vi "Moving Average.vi"(9 "New Value":dbl, 10 "# of Previous Elements":u64, 11 "Previous Average":dbl) -> (2 "Average":dbl)   [LabVIEW 2016]
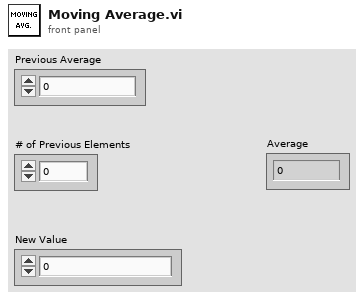
[diagram p1: front panel]
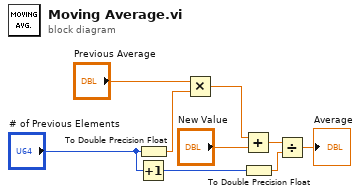
[diagram p0: block diagram]
diagram:
  n1 = Increment(x="# of Previous Elements") -> (x+1=w2:u64)
  n2 = To Double Precision Float(number="# of Previous Elements") -> (double precision float=w3:dbl)
  n3 = Multiply(x="Previous Average", y=w3) -> (x*y=w8:dbl)
  n4 = Add(x=w8, y="New Value") -> (x+y=w6:dbl)
  n5 = To Double Precision Float(number=w2) -> (double precision float=w1:dbl)
  n6 = Divide(x=w6, y=w1) -> (x/y=→"Average":dbl)
